vi "Trial Counter.vi"(11 "Input Path":path) -> (3 "Trial Number":i32)   [LabVIEW 2020, in "CollectionSupport.lvlib"]
uses:
  CollectionSupport.lvlib
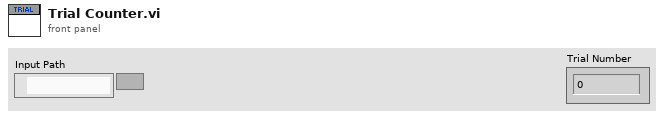
[diagram p1: front panel]
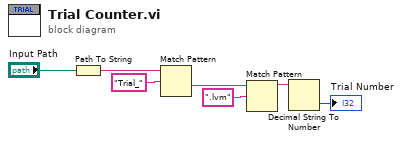
[diagram p0: block diagram]
diagram:
  n1 = Path To String(path="Input Path") -> (string=w5:string)
  n2 = Match Pattern(string=w5, regular expression="Trial_") -> (after substring=w3:string)  [unwired: 1 in, 3 out]
  n3 = Match Pattern(string=w3, regular expression=".lvm") -> (before substring=w2:string)  [unwired: 1 in, 3 out]
  n4 = Decimal String To Number(string=w2) -> (number=→"Trial Number":i32)  [unwired: 2 in, 1 out]
